vi "IntakeMain.vi"(6 "Error In":errorcluster, 7 "Reverse":bool, 8 "Forward":bool, 9 "Control Mode":enum16{"Open", "Control"}(ring)) -> (0 "Error Out":errorcluster)   [LabVIEW 2016]
uses:
  <vilib>/Rock Robotics/WPI/Relay/WPI_RelayValue.ctl
  <vilib>/Rock Robotics/SystemInterfaces/DIO/FPGA_DIORelayChannel.ctl
  <vilib>/Rock Robotics/WPI/Relay/WPI_RelayDirection.ctl
panel:
  # "Intake Control Main VI\nFRC Team 34"
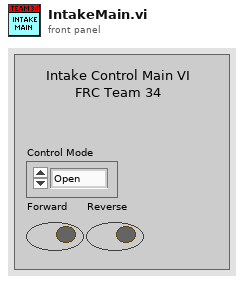
[diagram p1: front panel]
types:
  T1 = typedef "WPI_RelayValue.ctl" = enum16{"Off", "On", "Forward", "Reverse"}
  T2 = typedef "WPI_RelayDirection.ctl" = enum16{"Both directions", "Forward only", "Reverse only"}
  T3 = typedef "FPGA_DIORelayChannel.ctl" = enum8{"Relay 0", "Relay 1", "Relay 2", "Relay 3", "Invalid"}
  T4 = typedef "WPI_RelayDevRef.ctl" = cluster{"DevStatus":errorcluster, "Relay Channel":T3, "Relay Direction":T2}
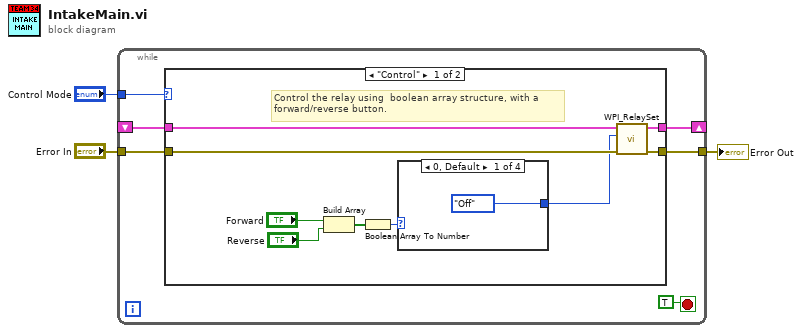
[diagram p0: block diagram]
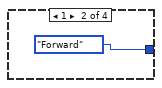
[diagram p2: hidden frame]
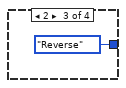
[diagram p3: hidden frame]
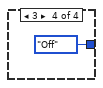
[diagram p4: hidden frame]
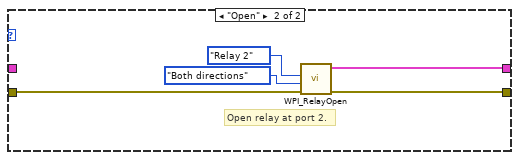
[diagram p5: hidden frame]
diagram:
  n1 = while {
    tunnel: "Control Mode" -> [w9]
    shift-right: [w7] -> _
    shift-left: _ -> [w6]
    tunnel: "Error In" -> [w5]
    tunnel: [w4] -> w2
    stop <- TRUE stop-if-true
    n2 = case shown="\"Control\"" w9 {
      tunnel: [w14 w25] -> w7
      tunnel: w6 -> [w11 _]
      tunnel: w5 -> [w12 w27]
      tunnel: [w13 w26] -> w4
      frame "Control" {
        # "Control the relay using  boolean array structure, with a \nforward/reverse button."
        n3 = Build Array("Forward", "Reverse") -> (w18:bool[])
        n4 = Boolean Array To Number(Boolean array=w18) -> (number=w15:u32)
        n5 = case shown="0, Default" w15 {
          tunnel: [WPI_RelayValue."Off" ("RelayValue") WPI_RelayValue."Forward" ("RelayValue") WPI_RelayValue."Reverse" ("RelayValue") WPI_RelayValue."Off" ("RelayValue")] -> w10
          frame 0, Default {
          }
          frame 1 {
          }
          frame 2 {
          }
          frame 3 {
          }
        }
        n6 = call <vilib>:"WPI_RelaySet.vi"("error in (no error)"=w12, "RelayValue"=w10, "RelayDevRef"=w11) -> ("error out"=w13:errorcluster, "RelayDevRef"=w14:T4)  [unwired: 7 in]
      }
      frame "Open" {
        # "Open relay at port 2."
        n7 = call <vilib>:"WPI_RelayOpen.vi"("error in (no error)"=w27, "Relay Direction"=WPI_RelayDirection."Both directions", "Relay Channel"=FPGA_DIORelayChannel."Relay 2") -> ("error out"=w26:errorcluster, "RelayDevRef"=w25:T4)  [unwired: 7 in]
      }
    }
  }
  "Error Out" <- w2
